vi "Queue.Initialization.vi"(8 "error in (no error)":errorcluster, 11 "queueName":string) -> (0 "error out":errorcluster)   [LabVIEW 2019]
uses:
  QueueMessage.ctl
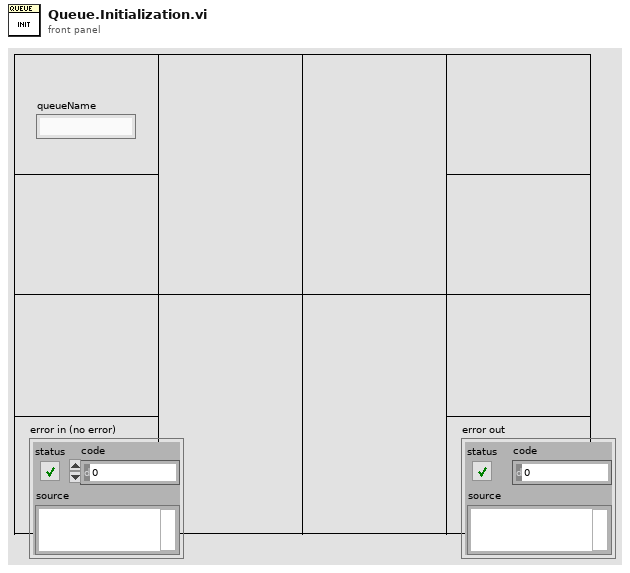
[diagram p1: front panel]
types:
  T1 = typedef "QueueMessage.ctl" = cluster{"message":string, "data":variant}
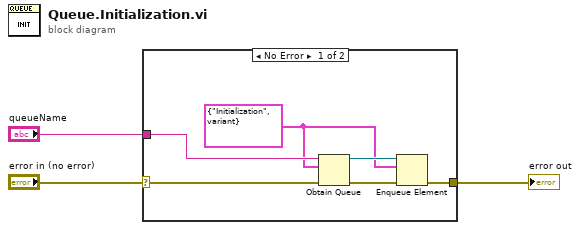
[diagram p0: block diagram]
diagram:
  n1 = case shown="No Error" "error in (no error)" {
    selector: "error in (no error)" -> [w6 w10]
    tunnel: "queueName" -> [w8 _]
    tunnel: [w9 w10] -> w2
    frame No Error {
      w4 = T1 {"message"="Initialization", "data"=variant} ("QueueMessage")
      n2 = Obtain Queue(name (unnamed)=w8, element data type=w4, error in (no error)=w6) -> (queue out=w7:refnum<queue>, error out=w5:errorcluster)  [unwired: 2 in, 1 out]
      n3 = Enqueue Element(queue=w7, element=w4, error in (no error)=w5) -> (error out=w9:errorcluster)  [unwired: 1 in, 2 out]
    }
    frame Error {
    }
  }
  "error out" <- w2
